vi "Serial Number Generator.vi"() -> (0 "UUT Serial #":string)   [LabVIEW 2012]
panel:
  out "Number 5":string
  out "Number 6":string
  out "Number 7":string
  out "Number 4":string
  out "Number 3":string
  out "Number 2":string
  out "Letter 4":string
  out "Letter 3":string
  out "Letter 2":string
  out "Letter":string
  out "Number":string
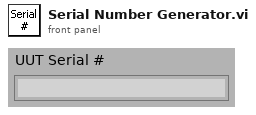
[diagram p1: front panel]
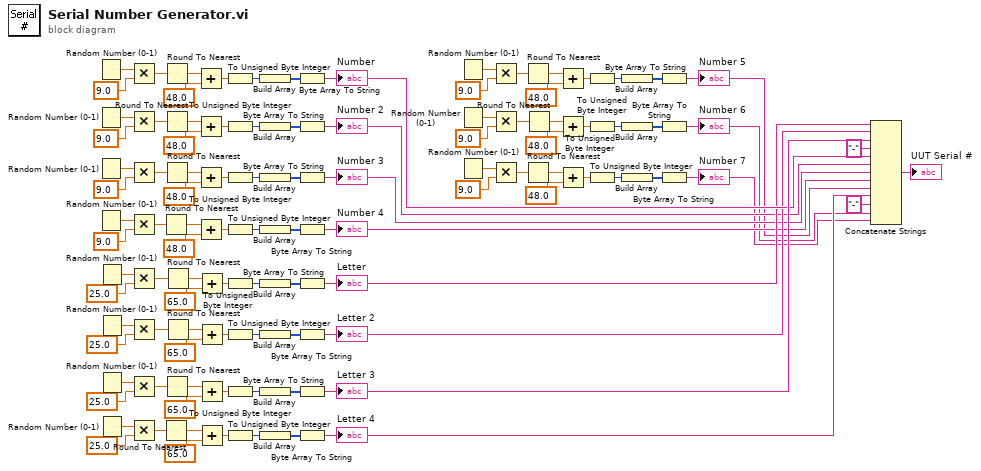
[diagram p0: block diagram]
diagram:
  n1 = Random Number (0-1)() -> (number: 0 to 1=w1:dbl)
  n2 = Random Number (0-1)() -> (number: 0 to 1=w59:dbl)
  n3 = Random Number (0-1)() -> (number: 0 to 1=w51:dbl)
  n4 = Random Number (0-1)() -> (number: 0 to 1=w44:dbl)
  n5 = Random Number (0-1)() -> (number: 0 to 1=w98:dbl)
  n6 = Random Number (0-1)() -> (number: 0 to 1=w79:dbl)
  n7 = Random Number (0-1)() -> (number: 0 to 1=w78:dbl)
  n8 = Random Number (0-1)() -> (number: 0 to 1=w64:dbl)
  n9 = Multiply(x=w1, y=9.0) -> (x*y=w95:dbl)
  n10 = Multiply(x=w59, y=9.0) -> (x*y=w61:dbl)
  n11 = Multiply(x=w51, y=9.0) -> (x*y=w53:dbl)
  n12 = Multiply(x=w44, y=9.0) -> (x*y=w42:dbl)
  n13 = Multiply(x=w98, y=25.0) -> (x*y=w94:dbl)
  n14 = Multiply(x=w79, y=25.0) -> (x*y=w81:dbl)
  n15 = Multiply(x=w78, y=25.0) -> (x*y=w76:dbl)
  n16 = Multiply(x=w64, y=25.0) -> (x*y=w66:dbl)
  n17 = Round To Nearest(number=w42) -> (nearest integer value=w9:dbl)
  n18 = Round To Nearest(number=w66) -> (nearest integer value=w5:dbl)
  n19 = Round To Nearest(number=w95) -> (nearest integer value=w12:dbl)
  n20 = Round To Nearest(number=w61) -> (nearest integer value=w11:dbl)
  n21 = Round To Nearest(number=w53) -> (nearest integer value=w10:dbl)
  n22 = Round To Nearest(number=w76) -> (nearest integer value=w6:dbl)
  n23 = Round To Nearest(number=w94) -> (nearest integer value=w8:dbl)
  n24 = Round To Nearest(number=w81) -> (nearest integer value=w7:dbl)
  n25 = Add(x=w12, y=48.0) -> (x+y=w91:dbl)
  n26 = Add(x=w11, y=48.0) -> (x+y=w63:dbl)
  n27 = Add(x=w10, y=48.0) -> (x+y=w55:dbl)
  n28 = Add(x=w9, y=48.0) -> (x+y=w40:dbl)
  n29 = Add(x=w8, y=65.0) -> (x+y=w87:dbl)
  n30 = Add(x=w7, y=65.0) -> (x+y=w86:dbl)
  n31 = Add(x=w6, y=65.0) -> (x+y=w72:dbl)
  n32 = Add(x=w5, y=65.0) -> (x+y=w71:dbl)
  n33 = To Unsigned Byte Integer(number=w91) -> (unsigned 8bit integer=w100:u8)
  n34 = To Unsigned Byte Integer(number=w63) -> (unsigned 8bit integer=w57:u8)
  n35 = To Unsigned Byte Integer(number=w55) -> (unsigned 8bit integer=w49:u8)
  n36 = To Unsigned Byte Integer(number=w40) -> (unsigned 8bit integer=w46:u8)
  n37 = To Unsigned Byte Integer(number=w87) -> (unsigned 8bit integer=w89:u8)
  n38 = To Unsigned Byte Integer(number=w86) -> (unsigned 8bit integer=w84:u8)
  n39 = To Unsigned Byte Integer(number=w72) -> (unsigned 8bit integer=w74:u8)
  n40 = To Unsigned Byte Integer(number=w71) -> (unsigned 8bit integer=w69:u8)
  n41 = Build Array(w100) -> (w101:u8[])
  n42 = Build Array(w57) -> (w56:u8[])
  n43 = Build Array(w49) -> (w48:u8[])
  n44 = Build Array(w46) -> (w47:u8[])
  n45 = Build Array(w89) -> (w88:u8[])
  n46 = Build Array(w84) -> (w85:u8[])
  n47 = Build Array(w74) -> (w73:u8[])
  n48 = Build Array(w69) -> (w70:u8[])
  n49 = Byte Array To String(unsigned byte array=w101) -> (string=w99:string)
  "Number" <- w99
  n50 = Byte Array To String(unsigned byte array=w56) -> (string=w58:string)
  "Number 2" <- w58
  n51 = Byte Array To String(unsigned byte array=w48) -> (string=w50:string)
  "Number 3" <- w50
  n52 = Byte Array To String(unsigned byte array=w47) -> (string=w45:string)
  "Number 4" <- w45
  n53 = Byte Array To String(unsigned byte array=w88) -> (string=w90:string)
  "Letter" <- w90
  n54 = Byte Array To String(unsigned byte array=w85) -> (string=w83:string)
  "Letter 2" <- w83
  n55 = Byte Array To String(unsigned byte array=w73) -> (string=w102:string)
  "Letter 3" <- w102
  n56 = Byte Array To String(unsigned byte array=w70) -> (string=w68:string)
  "Letter 4" <- w68
  n57 = Random Number (0-1)() -> (number: 0 to 1=w21:dbl)
  n58 = Random Number (0-1)() -> (number: 0 to 1=w30:dbl)
  n59 = Random Number (0-1)() -> (number: 0 to 1=w36:dbl)
  n60 = Multiply(x=w21, y=9.0) -> (x*y=w23:dbl)
  n61 = Multiply(x=w30, y=9.0) -> (x*y=w28:dbl)
  n62 = Multiply(x=w36, y=9.0) -> (x*y=w35:dbl)
  n63 = Round To Nearest(number=w23) -> (nearest integer value=w4:dbl)
  n64 = Round To Nearest(number=w35) -> (nearest integer value=w2:dbl)
  n65 = Round To Nearest(number=w28) -> (nearest integer value=w3:dbl)
  n66 = Add(x=w4, y=48.0) -> (x+y=w25:dbl)
  n67 = Add(x=w3, y=48.0) -> (x+y=w26:dbl)
  n68 = Add(x=w2, y=48.0) -> (x+y=w34:dbl)
  n69 = To Unsigned Byte Integer(number=w25) -> (unsigned 8bit integer=w19:u8)
  n70 = To Unsigned Byte Integer(number=w26) -> (unsigned 8bit integer=w32:u8)
  n71 = To Unsigned Byte Integer(number=w34) -> (unsigned 8bit integer=w38:u8)
  n72 = Build Array(w19) -> (w18:u8[])
  n73 = Build Array(w32) -> (w33:u8[])
  n74 = Build Array(w38) -> (w39:u8[])
  n75 = Byte Array To String(unsigned byte array=w18) -> (string=w20:string)
  "Number 5" <- w20
  n76 = Byte Array To String(unsigned byte array=w33) -> (string=w31:string)
  "Number 6" <- w31
  n77 = Byte Array To String(unsigned byte array=w39) -> (string=w37:string)
  "Number 7" <- w37
  n78 = Concatenate Strings(w90, w83, w102, "-" ("Substring"), w99, w58, w50, w45, w20, w68, "-" ("Substring"), w31, w37) -> (→"UUT Serial #":string)
